vi "SPI Flash Erase Chip.vi"(10 "SPIIndex":i32, 11 "DevHandle":i32) -> (3 "function return":i32)   [LabVIEW 2010, in "usb2spi.lvlib"]
doc: "int WINAPI SPI_FlashEraseChip(int DevHandle,int SPIIndex);"
uses:
  usb2spi.lvlib
  USB2XXX/trunk/USB2XXX/USB2XXX/vs2010/Release/USB2XXX.dll
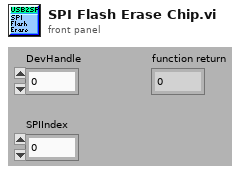
[diagram p1: front panel]
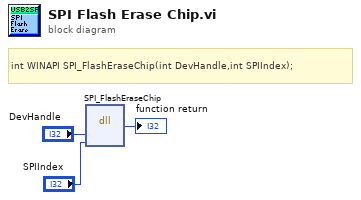
[diagram p0: block diagram]
diagram:
  # "int WINAPI SPI_FlashEraseChip(int DevHandle,int SPIIndex);"
  n1 = dll-call lib="E:/OtherWork/STM32/USB2XXX/trunk/USB2XXX/USB2XXX/vs2010/Release/USB2XXX.*" fn="SPI_FlashEraseChip"("DevHandle"="DevHandle", "SPIIndex"="SPIIndex") -> (→"function return":i32)  [unwired: 5 in, 2 out]
